vi "Team Move.vi"(4 "MIA?[p]":bool[](array[boolean]), 6 "Confirmed?[p]":bool[](array[boolean]), 7 "Move Cnt":i32, 8 "error in (no error)":errorcluster, 9 "Player[p] in":T1[](array[typedef]), 10 "p[x][y]":i32[][](array[numeric]), 11 "TeamEffort in":refnum<class "TeamEffort.lvclass">) -> (0 "error out":errorcluster, 1 "Player[p] out":T1[](array[typedef]), 3 "TeamEffort out":refnum<class "TeamEffort.lvclass">)   [LabVIEW 2015, in "TeamEffort.lvclass"]
uses:
  TeamEffort.lvclass
  private/Player Cluster.ctl
  Square/Square.lvclass
  Team Move Input.ctl
  Type Defs/Action Enum.ctl
  Team Move Output.ctl
  Type Defs/Direction Enum.ctl
  Type Defs/SB Type Defs.lvlib
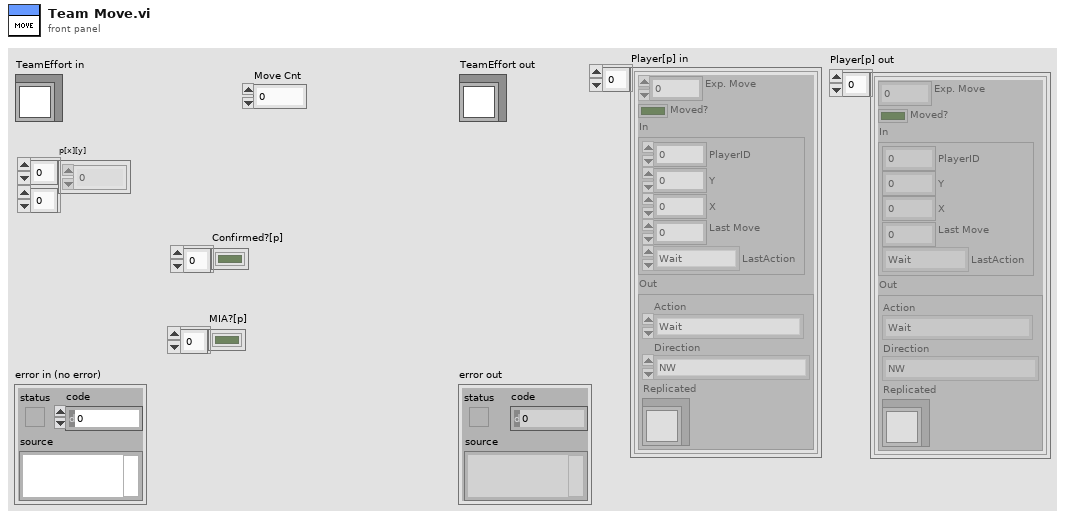
[diagram p1: front panel]
types:
  T1 = typedef "TeamEffort.lvclass/Player Cluster.ctl" = cluster{"Exp. Move":i32, "Moved?":bool, "In":T2, "Out":T4}
  T2 = typedef "TeamEffort.lvclass/Team Move Input.ctl" = cluster{"PlayerID":i32, "Y":i32, "X":i32, "Last Move":i32, "LastAction":T3}
  T3 = typedef "SB Type Defs.lvlib/Action Enum.ctl" = enum16{"Wait", "Move", "Attack", "Replicate"}
  T4 = typedef "TeamEffort.lvclass/Team Move Output.ctl" = cluster{"Action":T3, "Direction":T5, "Replicated":refnum<class "Square.lvclass">}
  T5 = typedef "SB Type Defs.lvlib/Direction Enum.ctl" = enum16{"NW", "N", "NE", "E", "SE", "S", "SW", "W"}
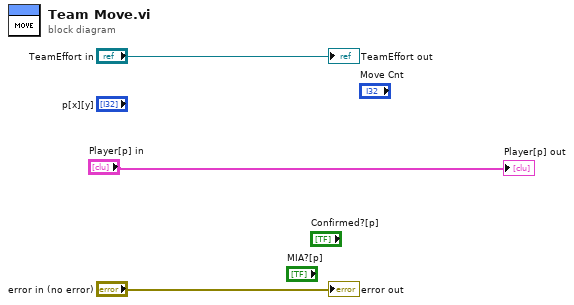
[diagram p0: block diagram]
diagram:
  "error out" <- "error in (no error)"
  "TeamEffort out" <- "TeamEffort in"
  "Player[p] out" <- "Player[p] in"
